vi "Configure Modulation (Frequency).vi"(0 "VISA resource name":refnum<visa-resource-name>, 1 "FM Source (0: Internal)":i32(ring) items=["Internal", "External", "CH1", "CH2"], 2 "Modulation Function (0: Sine)":i32(ring) items=["Sine", "Square", "Triangle", "Ramp", "NRamp", "Noise", "PRBS", "Arbitrary"], 5 "Channel (1: 1)":i32(ring)=1 items=["1"=1, "2"=2], 7 "Enable Frequency Modulation(T: Enable)":bool=TRUE, 11 "error in (no error)":errorcluster, 12 "Peak Deviation Value (100 Hz)":dbl=100.0, 13 "Modulation Frequency (100 Hz)":dbl=100.0, 14 "Sample Rate (40000 Sa/s)":dbl=40000.0) -> (4 "VISA resource name out":refnum<visa-resource-name>, 15 "error out":errorcluster)   [LabVIEW 2015, in "Agilent 3352X Series.lvlib"]
doc: "Configures and enables frequency modulation (FM). In FM, the frequency of the carrier is varied by the frequency of the modulating waveform. \n\n<b>Note</b>: \n(1) When enabling this mode, all other modes will be turned off.\n(2) The carrier waveform shape and parameters are set by the Configure Standard Waveform VI, Configure PRBS Waveform VI, or Configure Pulse Waveform VI\n(3) You can select a sine, square, ramp, pulse, or PRBS waveform for the carrier (noise, arbitrary, and DC are not allowed)."
uses:
  <instrlib>/Agilent 3352X Series/Agilent 3352X Series.lvlib
panel:
  # "Internal FM Settings"
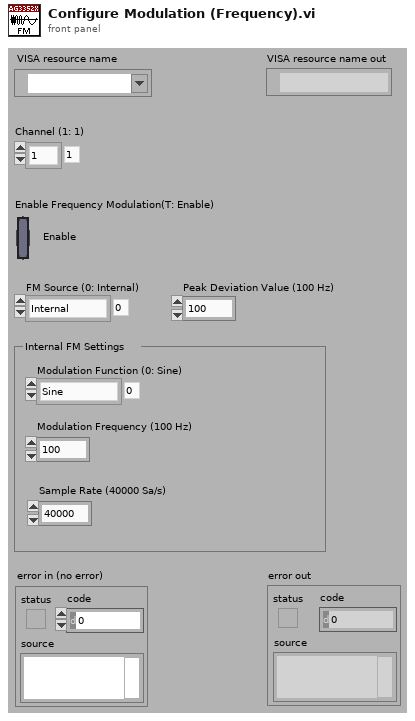
[diagram p1: front panel]
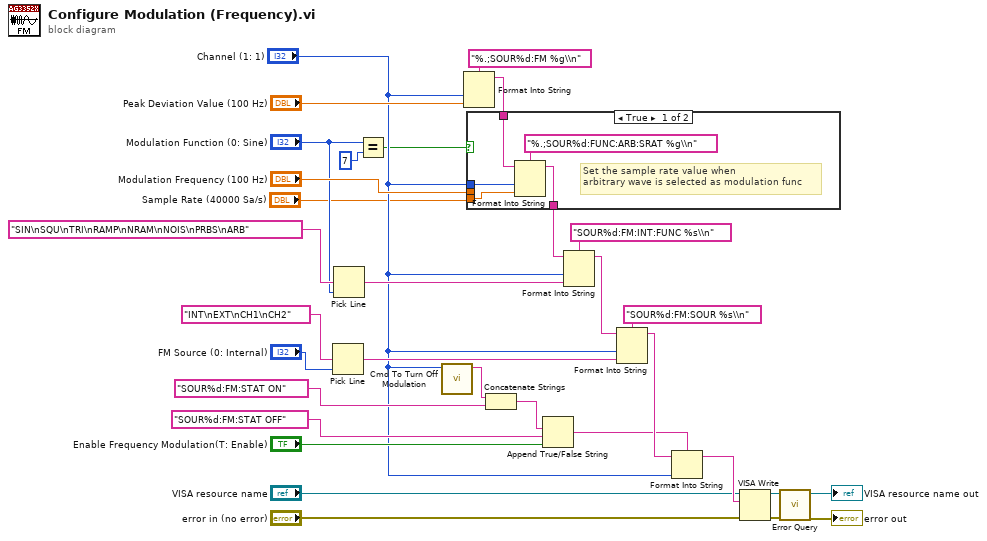
[diagram p0: block diagram]
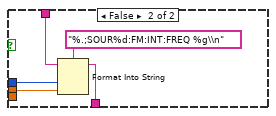
[diagram p2: hidden frame]
diagram:
  n1 = Pick Line(multi-line string="INT\nEXT\nCH1\nCH2", line index="FM Source (0: Internal)") -> (output string=w26:string)  [unwired: 1 out]
  n2 = Pick Line(multi-line string="SIN\nSQU\nTRI\nRAMP\nNRAM\nNOIS\nPRBS\nARB", line index="Modulation Function (0: Sine)") -> (output string=w15:string)  [unwired: 1 out]
  n3 = Equal?(x="Modulation Function (0: Sine)", y=u16 7) -> (x = y?=w3:bool)
  n4 = call <instrlib>:"Cmd To Turn Off Modulation.vi"("Channel (1: 1)"="Channel (1: 1)") -> ("Cmd String"=w11:string)  [unwired: 10 out]
  n5 = Format Into String(format string="%.;SOUR%d:FM %g\\n", "Channel (1: 1)", "Peak Deviation Value (100 Hz)") -> (resulting string=w14:string)  [unwired: 2 in, 1 out]
  n6 = case shown="True" w3 {
    tunnel: w14 -> [w36 w42]
    tunnel: "Modulation Frequency (100 Hz)" -> [_ w41]
    tunnel: [w37 w40] -> w12
    tunnel: "Channel (1: 1)" -> [w35 w38]
    tunnel: "Sample Rate (40000 Sa/s)" -> [w33 _]
    frame True {
      # "Set the sample rate value when\narbitrary wave is selected as modulation func"
      n7 = Format Into String(format string="%.;SOUR%d:FUNC:ARB:SRAT %g\\n", initial string=w36, w35, w33) -> (resulting string=w37:string)  [unwired: 1 in, 1 out]
    }
    frame False {
      n8 = Format Into String(format string="%.;SOUR%d:FM:INT:FREQ %g\\n", initial string=w42, w38, w41) -> (resulting string=w40:string)  [unwired: 1 in, 1 out]
    }
  }
  n9 = Concatenate Strings(w11, "SOUR%d:FM:STAT ON") -> (w8:string)
  n10 = Append True/False String(1:"Enable Frequency Modulation(T: Enable)", 2:"SOUR%d:FM:STAT OFF", 3:w8) -> (0:w9:string)  [unwired: 1 out]
  n11 = Format Into String(format string="SOUR%d:FM:INT:FUNC %s\\n", initial string=w12, "Channel (1: 1)", w15) -> (resulting string=w28:string)  [unwired: 1 in, 1 out]
  n12 = Format Into String(format string="SOUR%d:FM:SOUR %s\\n", initial string=w28, "Channel (1: 1)", w26) -> (resulting string=w23:string)  [unwired: 1 in, 1 out]
  n13 = Format Into String(format string=w9, initial string=w23, "Channel (1: 1)") -> (resulting string=w22:string)  [unwired: 1 in, 1 out]
  n14 = VISA Write(VISA resource name="VISA resource name", write buffer=w22, error in (no error)="error in (no error)") -> (VISA resource name out=w19:refnum<visa-resource-name>, error out=w18:errorcluster)  [unwired: 1 out]
  n15 = call <instrlib>:"Error Query.vi"("error in (no error)"=w18, "VISA resource name"=w19) -> ("error out"=→"error out":errorcluster, "VISA resource name out"=→"VISA resource name out":refnum<visa-resource-name>)  [unwired: 8 out]
